vi "Create AI task.vi"(4 "Variables":T1) -> (1 "Variables out":T1)   [LabVIEW 2020]
uses:
  Constants.ctl
  <resource>/objmgr/daqmx.rc
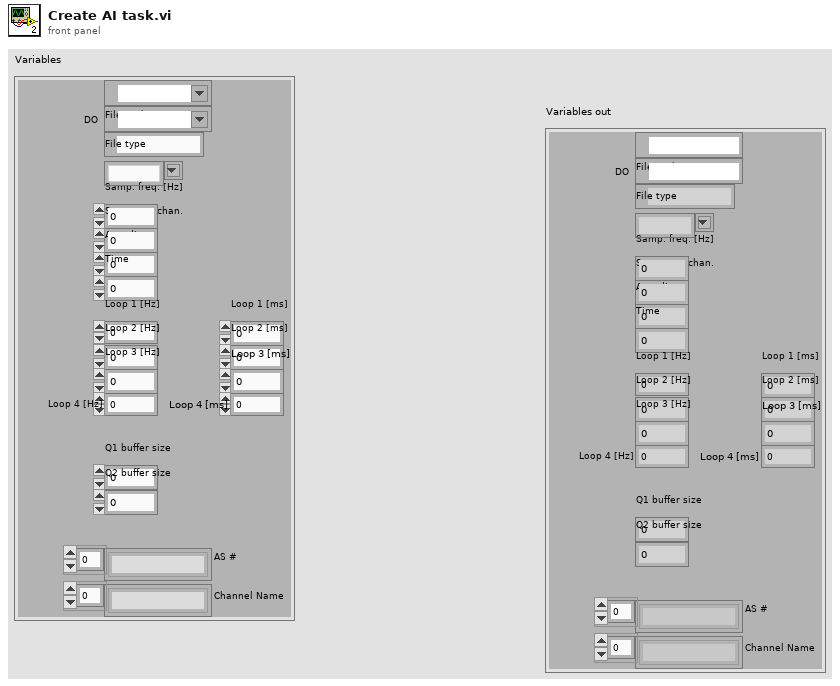
[diagram p1: front panel]
types:
  T1 = typedef "Constants.ctl" = cluster{"Time":u16, "Samp. freq. [Hz]":dbl, "Samp. per chan.":i32, "Avg. div.":i32, "File path":path, "AI":refnum<k21>, "Loop 1 [Hz]":dbl, "Loop 2 [Hz]":dbl, "Loop 3 [Hz]":dbl, "Loop 1 [ms]":dbl, "Loop 2 [ms]":dbl, "Loop 3 [ms]":dbl, "Q1 buffer size":i32, "Q2 buffer size":i32, "File type":string, "Loop 4 [Hz]":dbl, "Loop 4 [ms]":dbl, "Channel Name":string[], "AS #":string[], "DO":refnum<k21>}
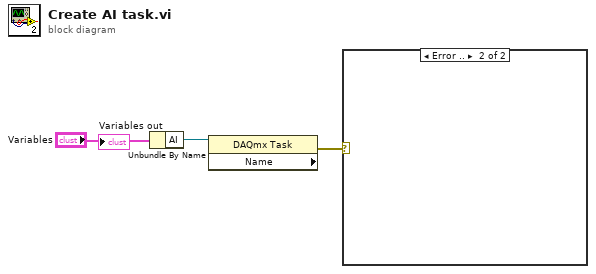
[diagram p0: block diagram]
diagram:
  n1 = Unbundle By Name("Variables") -> ("AI"=w2:refnum<k21>)
  n2 = property class="DAQmx Task" props=["Name"](reference=w2) -> (error out=w1:errorcluster)  [unwired: 1 in, 2 out]
  n3 = case shown="Error .." w1 {
    frame No Error {
    }
    frame Error {
    }
  }
  "Variables out" <- "Variables"
